vi "Sender.vi"() -> ()   [LabVIEW 2019]
panel:
  out "Humdity":dbl
  out "Temperature":dbl
  in  "stop":bool
  # "Sender"
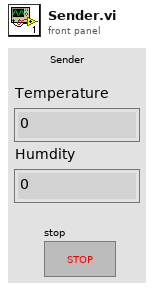
[diagram p1: front panel]
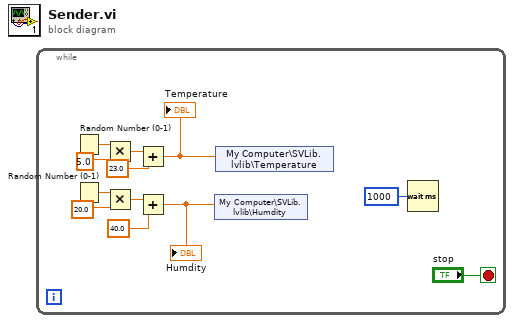
[diagram p0: block diagram]
diagram:
  n1 = while {
    stop <- "stop" stop-if-true
    n2 = Random Number (0-1)() -> (number: 0 to 1=w12:dbl)
    n3 = Random Number (0-1)() -> (number: 0 to 1=w4:dbl)
    n4 = Multiply(x=w12, y=5.0) -> (x*y=w10:dbl)
    n5 = Multiply(x=w4, y=20.0) -> (x*y=w6:dbl)
    n6 = Add(x=w10, y=23.0) -> (x+y=w8:dbl)
    "Temperature" <- w8
    n7 = Add(x=w6, y=40.0) -> (x+y=w3:dbl)
    "Humdity" <- w3
    n8 = shared-variable "My Computer\\SVLib.lvlib\\Humdity"(w3) -> ()  [unwired: 1 in, 1 out]
    n9 = shared-variable "My Computer\\SVLib.lvlib\\Temperature"(w8) -> ()  [unwired: 1 in, 1 out]
    n10 = Wait (ms)(milliseconds to wait=u32 1000) -> ()  [unwired: 1 out]
  }
